vi "ButtonEvents.vi"(11 "UiDefinition":T1) -> ()   [LabVIEW 2020]
uses:
  UIReferences.ctl
  D:/LabviewDXFViewer/LabviewDXFViewer/bin/Release/LabviewDXFViewer.exe
  LabviewDXFViewer/bin/Release/LabviewDXFViewer.exe
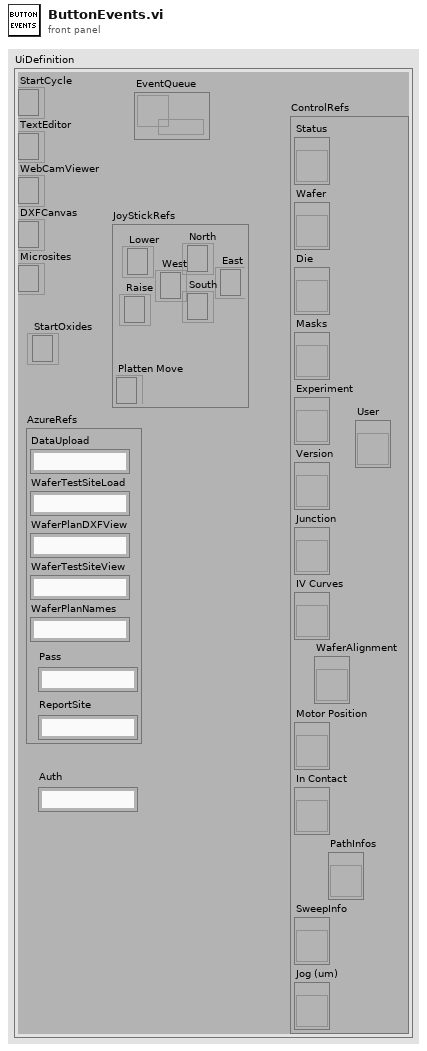
[diagram p1: front panel]
types:
  T1 = typedef "UIReferences.ctl" = cluster{"StartCycle":refnum<k24>, "TextEditor":refnum<k24>, "WebCamViewer":refnum<k24>, "DXFCanvas":refnum<k24>, "Microsites":refnum<k24>, "JoyStickRefs":cluster{"North":refnum<k24>, "Lower":refnum<k24>, "Raise":refnum<k24>, "Platten Move":refnum<k24>, "West":refnum<k24>, "East":refnum<k24>, "South":refnum<k24>}, "AzureRefs":cluster{"DataUpload":string, "WaferTestSiteLoad":string, "WaferPlanDXFView":string, "WaferTestSiteView":string, "WaferPlanNames":string, "Pass":string, "ReportSite":string}, "ControlRefs":cluster{"Status":refnum<vi>, "Wafer":refnum<vi>, "Die":refnum<vi>, "Masks":refnum<vi>, "Experiment":refnum<vi>, "Version":refnum<vi>, "Junction":refnum<vi>, "IV Curves":refnum<vi>, "Motor Position":refnum<vi>, "In Contact":refnum<vi>, "SweepInfo":refnum<vi>, "Jog (um)":refnum<vi>, "PathInfos":refnum<vi>, "User":refnum<vi>, "WaferAlignment":refnum<vi>}, "EventQueue":refnum<queue>, "StartOxides":refnum<k24>, "Auth":string}
  T2 = cluster{"North":refnum<k24>, "Lower":refnum<k24>, "Raise":refnum<k24>, "Platten Move":refnum<k24>, "West":refnum<k24>, "East":refnum<k24>, "South":refnum<k24>}
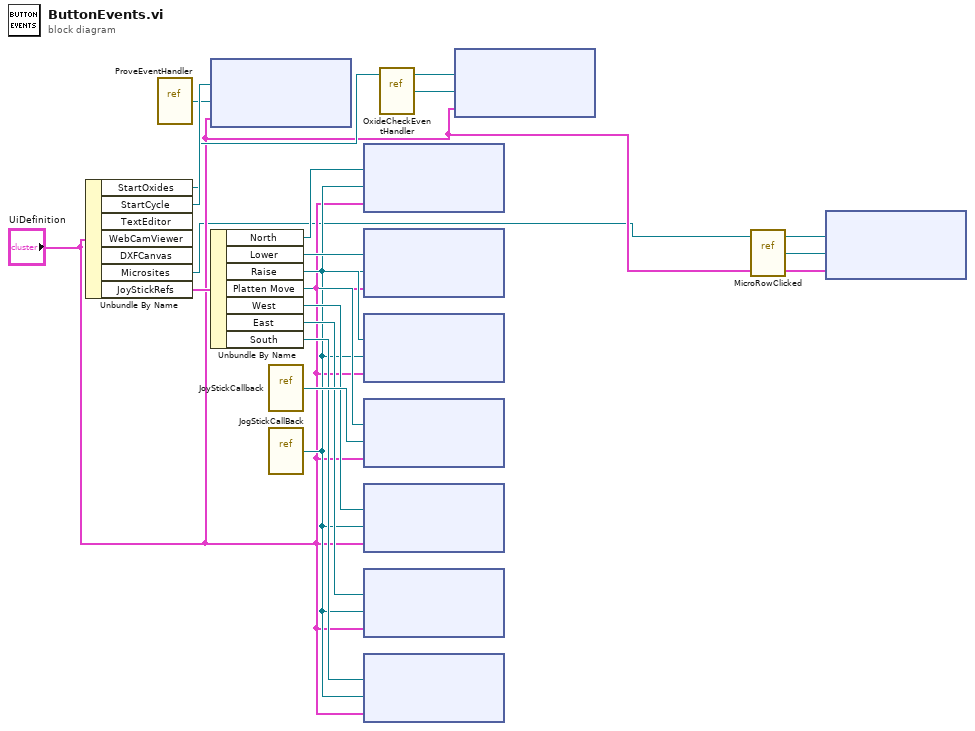
[diagram p0: block diagram]
diagram:
  n1 = Unbundle By Name("UiDefinition") -> ("StartOxides"=w5:refnum<k24>, "StartCycle"=w16:refnum<k24>, "Microsites"=w2:refnum<k24>, "JoyStickRefs"=w17:T2)  [unwired: 3 out]
  n2 = vi-ref "ProveEventHandler.vi"() -> ("vi reference"=w15:refnum<vi>)
  n3 = node(w16, w15, "UiDefinition") -> ()  [unwired: 2 in, 2 out]
  n4 = Unbundle By Name(w17) -> ("North"=w8:refnum<k24>, "Lower"=w12:refnum<k24>, "Raise"=w11:refnum<k24>, "Platten Move"=w14:refnum<k24>, "West"=w10:refnum<k24>, "East"=w9:refnum<k24>, "South"=w7:refnum<k24>)
  n5 = vi-ref "JoyStickCallback.vi"() -> ("vi reference"=w13:refnum<vi>)
  n6 = vi-ref "JogStickCallBack.vi"() -> ("vi reference"=w6:refnum<vi>)
  n7 = node(w8, w6, "UiDefinition") -> ()  [unwired: 2 in, 2 out]
  n8 = node(w12, w6, "UiDefinition") -> ()  [unwired: 2 in, 2 out]
  n9 = node(w11, w6, "UiDefinition") -> ()  [unwired: 2 in, 2 out]
  n10 = node(w14, w13, "UiDefinition") -> ()  [unwired: 2 in, 2 out]
  n11 = node(w10, w6, "UiDefinition") -> ()  [unwired: 2 in, 2 out]
  n12 = node(w9, w6, "UiDefinition") -> ()  [unwired: 2 in, 2 out]
  n13 = node(w7, w6, "UiDefinition") -> ()  [unwired: 2 in, 2 out]
  n14 = vi-ref "OxideCheckEventHandler.vi"() -> ("vi reference"=w4:refnum<vi>)
  n15 = node(w5, w4, "UiDefinition") -> ()  [unwired: 2 in, 2 out]
  n16 = vi-ref "MicroRowClicked.vi"() -> ("vi reference"=w1:refnum<vi>)
  n17 = node(w2, w1, "UiDefinition") -> ()  [unwired: 2 in, 2 out]
